vi "Read Device Labels.vi"(8 "error in (no error)":errorcluster, 11 "VoiceMeeterRemote in":refnum<class "VoiceMeeterRemote.lvclass">) -> (0 "error out":errorcluster, 1 "Output Labels":string[](array[string]), 2 "Input Labels":string[](array[string]), 3 "VoiceMeeterRemote out":refnum<class "VoiceMeeterRemote.lvclass">)   [LabVIEW 2022 SP3, in "VoiceMeeterRemote.lvlib" / "VoiceMeeterRemote.lvclass"]
doc: "Returns the labels that have been set for all of the inputs and outputs in Voicemeeter."
uses:
  VoiceMeeterRemote.lvclass
  VoiceMeeterRemote.lvclass/VoiceMeeterRemote.ctl
  VoiceMeeterRemote.lvlib
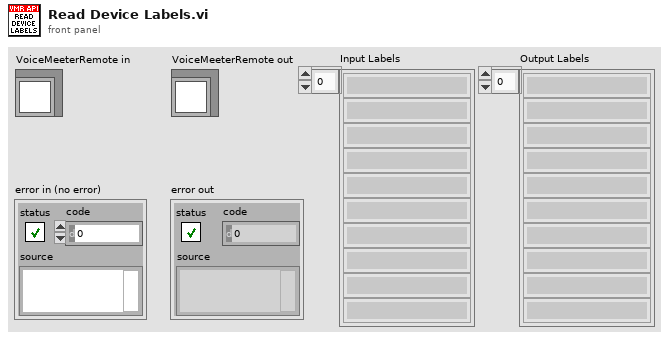
[diagram p1: front panel]
types:
  T1 = typedef "VoiceMeeterRemote.lvlib/Voicemeeter Type.ctl" = enum16{"Unknown", "Voicemeeter", "Banana", "Potato", "Potato x64"}
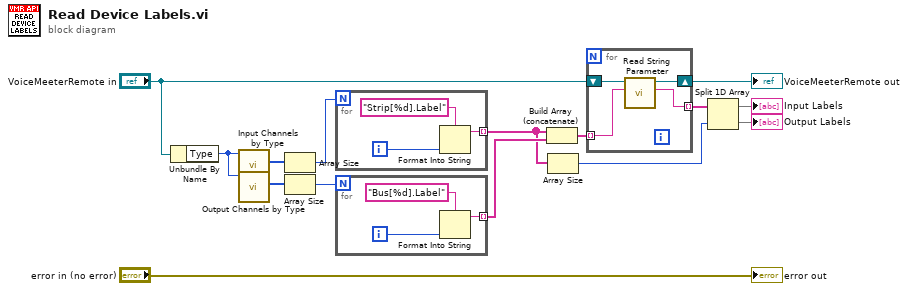
[diagram p0: block diagram]
diagram:
  n1 = Unbundle By Name("VoiceMeeterRemote in") -> ("Type"=w12:T1)
  n2 = call "Input Channels by Type.vi"("Voicemeeter Type"=w12) -> ("Channel Count"=w14:i32[])  [unwired: 10 in]
  n3 = call "Output Channels by Type.vi"("Voicemeeter Type"=w12) -> ("Channel Count"=w13:i32[])  [unwired: 10 in]
  n4 = Array Size(array=w14) -> (size(s)=w11:i32)
  n5 = Array Size(array=w13) -> (size(s)=w10:i32)
  n6 = for {
    N: w11 -> [_]
    tunnel: [w16] -> w5 mode=indexing
    i -> [w17]
    n7 = Format Into String(format string="Strip[%d].Label", w17) -> (resulting string=w16:string)  [unwired: 2 in, 1 out]
  }
  n8 = for {
    N: w10 -> [_]
    tunnel: [w19] -> w9 mode=indexing
    i -> [w20]
    n9 = Format Into String(format string="Bus[%d].Label", w20) -> (resulting string=w19:string)  [unwired: 2 in, 1 out]
  }
  n10 = Build Array (concatenate)(w5, w9) -> (w8:string[])
  n11 = Array Size(array=w5) -> (size(s)=w1:i32)
  n12 = for {
    tunnel: w8 -> [w24] mode=indexing
    shift-right: [w23] -> w6
    shift-left: "VoiceMeeterRemote in" -> [w25]
    tunnel: [w22] -> w4 mode=indexing
    n13 = call "Read String Parameter.vi"("Parameter Name"=w24, "VoiceMeeterRemote in"=w25) -> ("Value"=w22:string, "VoiceMeeterRemote out"=w23:refnum<class "VoiceMeeterRemote.lvclass">)  [unwired: 7 in, 1 out]
  }
  "VoiceMeeterRemote out" <- w6
  n14 = Split 1D Array(array=w4, index=w1) -> (first subarray=→"Input Labels":string[], second subarray=→"Output Labels":string[])
  "error out" <- "error in (no error)"
